vi "Read Time.vi"(8 "error in (no error)":errorcluster, 11 "TreeItemOpenMsg in":refnum<class "TreeItemOpenMsg.lvclass">) -> (0 "error out":errorcluster, 2 "Time":u32, 3 "TreeItemOpenMsg out":refnum<class "TreeItemOpenMsg.lvclass">)   [LabVIEW 2017, in "ActorEvents.lvlib" / "TreeItemOpenMsg.lvclass"]
uses:
  TreeItemOpenMsg.lvclass
  TreeItemOpenMsg.lvclass/TreeItemOpenMsg.ctl
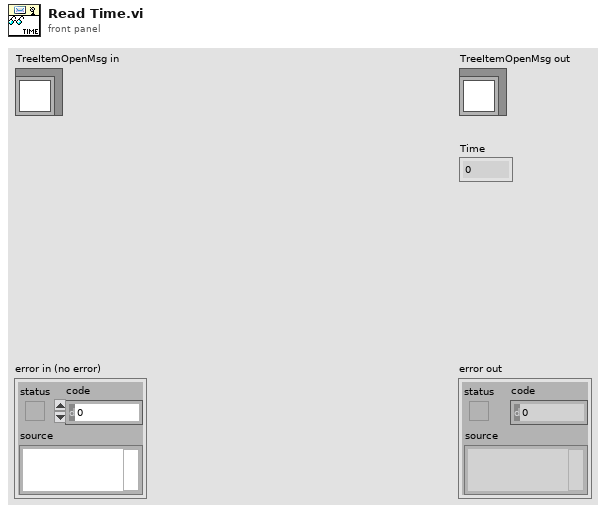
[diagram p1: front panel]
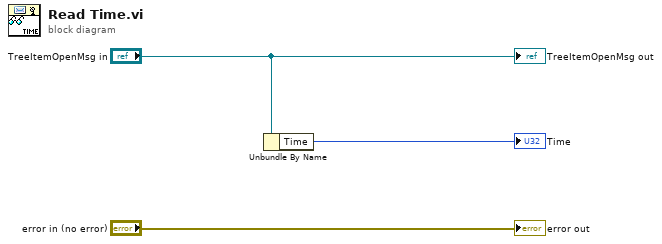
[diagram p0: block diagram]
diagram:
  n1 = Unbundle By Name("TreeItemOpenMsg in") -> ("Time"=→"Time":u32)
  "error out" <- "error in (no error)"
  "TreeItemOpenMsg out" <- "TreeItemOpenMsg in"
